vi "Read Output.vi"(8 "error in":errorcluster, 11 "VISA resource name":refnum<visa-resource-name>) -> (0 "error out":errorcluster, 1 "Actual Current Level (A)":dbl format="%.2g", 2 "Actual Voltage Level (V)":dbl format="%.2g", 3 "VISA resource name out":refnum<visa-resource-name>)   [LabVIEW 2024, in "IT-M3900C.lvlib"]
doc: "Returns the actual voltage level and actual current level for a desired channel."
uses:
  IT-M3900C.lvlib
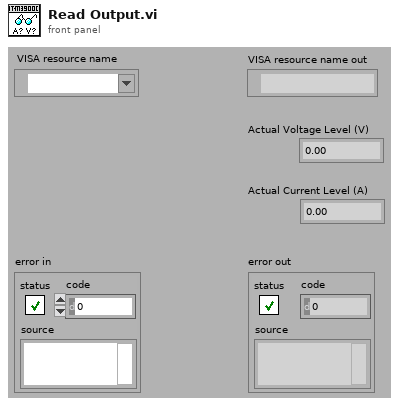
[diagram p1: front panel]
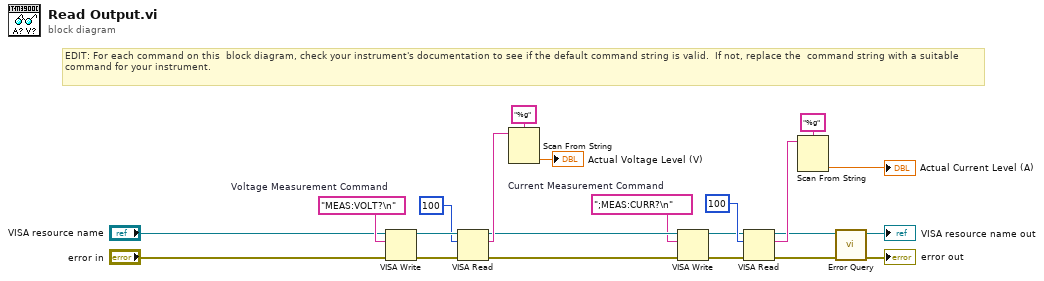
[diagram p0: block diagram]
diagram:
  w4 = ";MEAS:CURR?\n"  # Current Measurement Command
  w3 = "MEAS:VOLT?\n"  # Voltage Measurement Command
  # "EDIT: For each command on this  block diagram, check your instrument's documentation to see if the default command string is valid.  If not, replace the  command string with a suitable command for your instrument."
  n1 = VISA Write(VISA resource name="VISA resource name", write buffer=w3, error in (no error)="error in") -> (VISA resource name out=w21:refnum<visa-resource-name>, error out=w22:errorcluster)  [unwired: 1 out]
  n2 = VISA Read(VISA resource name=w21, byte count=u32 100, error in (no error)=w22) -> (VISA resource name out=w5:refnum<visa-resource-name>, read buffer=w16:string, error out=w6:errorcluster)  [unwired: 1 out]
  n3 = Scan From String(format string="%g", input string=w16) -> (output 1=→"Actual Voltage Level (V)":dbl)  [unwired: 3 in, 3 out]
  n4 = VISA Write(VISA resource name=w5, write buffer=w4, error in (no error)=w6) -> (VISA resource name out=w11:refnum<visa-resource-name>, error out=w10:errorcluster)  [unwired: 1 out]
  n5 = VISA Read(VISA resource name=w11, byte count=u32 100, error in (no error)=w10) -> (VISA resource name out=w8:refnum<visa-resource-name>, read buffer=w13:string, error out=w7:errorcluster)  [unwired: 1 out]
  n6 = Scan From String(format string="%g", input string=w13) -> (output 1=→"Actual Current Level (A)":dbl)  [unwired: 3 in, 3 out]
  n7 = call "Error Query.vi"("error in"=w7, "VISA resource name"=w8) -> ("error out"=→"error out":errorcluster, "VISA resource name out"=→"VISA resource name out":refnum<visa-resource-name>)  [unwired: 6 in, 2 out]
